vi "LatchBoolean.vi"(9 "Reset":bool, 10 "Set":bool, 11 "D":bool) -> (3 "Q":bool)   [LabVIEW 2019]
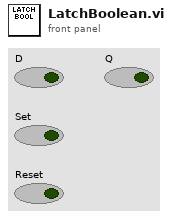
[diagram p1: front panel]
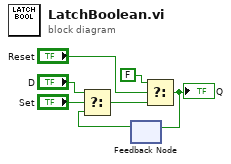
[diagram p0: block diagram]
diagram:
  n1 = feedback #1() -> (w4:bool)  [unwired: 1 in]
  n2 = Select(t="D", s="Set", f=w4) -> (s? t:f=w2:bool)
  n3 = Select(t=FALSE, s="Reset", f=w2) -> (s? t:f=w7:bool)
  "Q" <- w7
  n4 = feedback-in #1(w7) -> ()
